vi "Label_Ranking_Loss.vi"(7 "Type y_true":T1(ring), 8 "error in (no error)":errorcluster caption="entrée d'erreur (pas d'erreur)", 9 "y_score":string[][](array[string]), 10 "y_true":string[][](array[string]), 11 "label_ranking_loss":cluster{"sample_weight":dbl[]}) -> (0 "error out":errorcluster caption="sortie d'erreur", 3 "Score":string)   [LabVIEW 2020]
doc: "Compute Ranking loss measure\n\nCompute the average number of label pairs that are incorrectly ordered given y_score weighted by the size of the label set and the number of labels not in the label set.\n\nThis is similar to the error set size, but weighted by the number of relevant and irrelevant labels. The best performance is achieved with a ranking loss of zero.\n\n\n\nParameters : \n\n- y_true : array or sparse matrix, shape = [n_samples, n_labels]\nTrue binary labels in binary indicator format.\n\n- y_score : array, shape = [n_samples, n_labels]\nTarget scores, can either be probability estimates of the positive class, confidence values, or non-thresholded measure of decisions (as returned by “decision_function” on some classifiers).\n\n- sample_weight : array-like of shape (n_samples,), default=None\nSample weights.\n\nReturns : \n\n- loss : float"
uses:
  Label_Ranking_Loss.lvclass
panel:
  out "Label_Ranking_Loss.lvclass":refnum<class "Label_Ranking_Loss.lvclass">
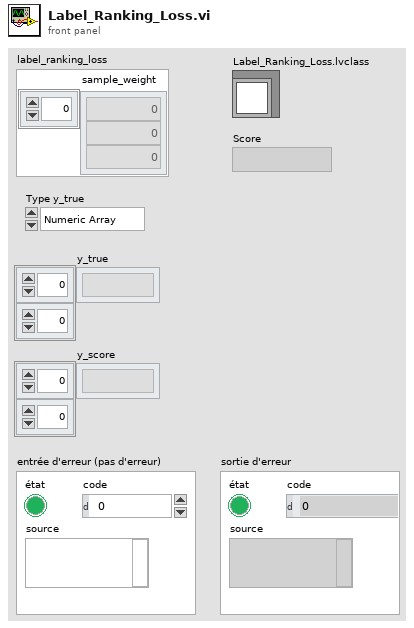
[diagram p1: front panel]
types:
  T1 = enum16{"Numeric Array", "String Array", "Sparse"}
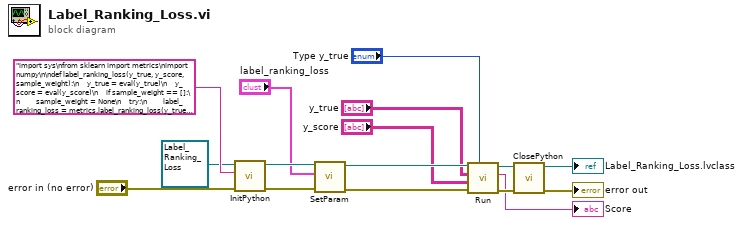
[diagram p0: block diagram]
diagram:
  n1 = call-dynamic "InitPython.vi"("error in (no error)"="error in (no error)", "Python Instruction"="import sys\nfrom sklearn import metrics\nimport numpy\n\ndef label_ranking_loss(y_true, y_score, sample_weight):\n    y_true = eval(y_true)\n    y_score = eval(y_score)\n    if sample_weight == []:\n        sample_weight = None\n    try:\n        label_ranking_loss = metrics.label_ranking_loss(y_true, y_score, sample_weight)\n        label_ranking_loss = label_ranking_loss.tolist()\n        return str(label_ranking_loss)\n    except:\n        erreur = sys.exc_info()\n        typerr = u\"%s\" % (erreur[0])\n        typerr = typerr[typerr.find(\"'\")+1:typerr.rfind(\"'\")]\n        msgerr = u\"%s\" % (erreur[1])\n        message = str('/!\\\\ {0} : {1}'. format(typerr,msgerr))\n        return message", "Scikit-learn en entrée"=refnum<class "Label_Ranking_Loss.lvclass"> refnum ("Label_Ranking_Loss.lvclass")) -> ("error out"=w11:errorcluster, "Scikit-learn en sortie"=w12:refnum<class "Label_Ranking_Loss.lvclass">)  [unwired: 7 in]
  n2 = call-dynamic "SetParam.vi"("error in (no error)"=w11, "label_ranking_loss"="label_ranking_loss", "Label_Ranking_Loss.lvclass"=w12) -> ("error out"=w8:errorcluster, "Label_Ranking_Loss.lvclass"=w9:refnum<class "Label_Ranking_Loss.lvclass">)  [unwired: 7 in]
  n3 = call-dynamic "Run.vi"("Type y_true"="Type y_true", "error in (no error)"=w8, "y_score"="y_score", "y_true"="y_true", "Label_Ranking_Loss.lvclass"=w9) -> ("error out"=w6:errorcluster, "String Data"=→"Score":string, "Label_Ranking_Loss.lvclass"=w7:refnum<class "Label_Ranking_Loss.lvclass">)  [unwired: 4 in]
  n4 = call-dynamic "ClosePython.vi"("error in (no error)"=w6, "Scikit-learn en entrée"=w7) -> ("error out"=→"error out":errorcluster, "Scikit-learn en sortie"=→"Label_Ranking_Loss.lvclass":refnum<class "Label_Ranking_Loss.lvclass">)  [unwired: 8 in]
